vi "Grab.vi"() -> ()   [LabVIEW 2013]
doc: "The Grab VI acquires images continuously and displays the images in an image control using high-level acquisition VIs. A grab is appropriate for high-speed applications in which you need to process only one image at a time."
uses:
  <vilib>/vision/driver/NI_Vision_Acquisition_Software.lvlib
panel:
  out "appended path":path
  in  "Camera Name":refnum<k21> caption="IMAQdx Session"
  out "Buffer Number":u32
  out "Image":T1(plugin-control)
  out "Frame Rate":dbl(knob) scale=0.0..100.0
  in  "Stop":bool
  # "Overview: Demonstrates how to acquire images continuously using a Grab acquisition.\nRequirements: Vision Acquisition Software\nInstructions: \n1. Select the Camera Name.\n2. Run the VI"
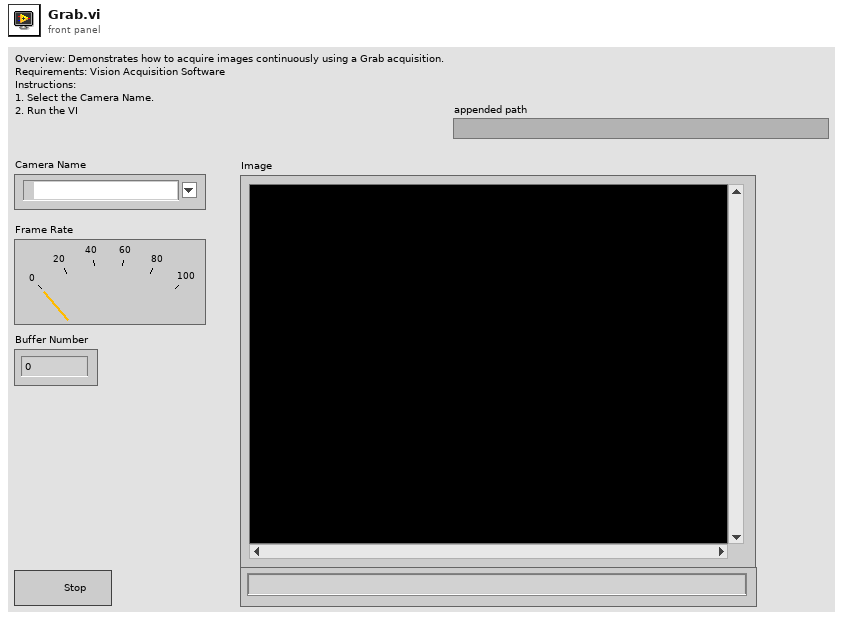
[diagram p1: front panel]
types:
  T1 = typedef "IMAQ Image.ctl" = refnum<image>
  T2 = typedef "IMAQdx.ctl" = refnum<k21>
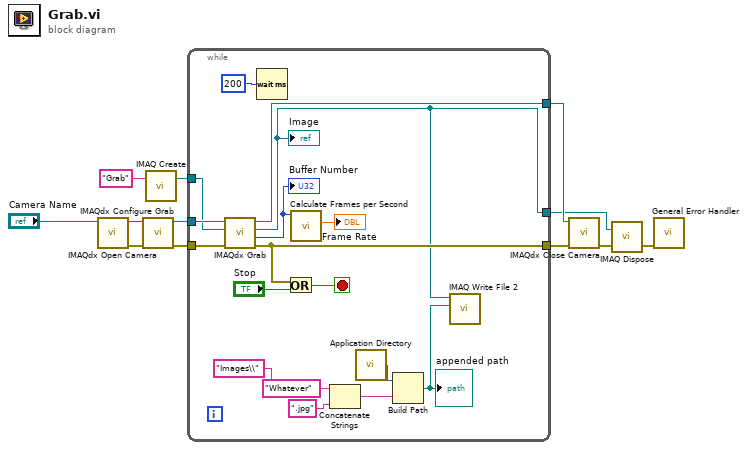
[diagram p0: block diagram]
diagram:
  n1 = call <vilib>:"IMAQdx Open Camera.vi"("Session In"="Camera Name") -> ("error out"=w7:errorcluster, "Session Out"=w6:T2)  [unwired: 2 in, 7 out]
  n2 = call <vilib>:"IMAQdx Configure Grab.vi"("error in"=w7, "Session In"=w6) -> ("error out"=w10:errorcluster, "Session Out"=w11:T2)  [unwired: 8 out]
  n3 = call "IMAQ Create"("Image Name"="Grab") -> ("New Image"=w12:T1)  [unwired: 3 in, 2 out]
  n4 = while {
    tunnel: [w24] -> w9
    tunnel: w10 -> [w26]
    tunnel: w11 -> [w27]
    tunnel: [w21] -> w8
    tunnel: w12 -> [w25]
    tunnel: [w20] -> w4
    stop <- w29 stop-if-true
    n5 = call <vilib>:"IMAQdx Grab.vi"("error in"=w26, "Image In"=w25, "Session In"=w27) -> ("error out"=w21:errorcluster, "Buffer Number Out"=w22:u32, "Image Out"=w20:T1, "Session Out"=w24:T2)  [unwired: 1 in, 4 out]
    "Image" <- w20
    "Buffer Number" <- w22
    n6 = Wait (ms)(milliseconds to wait=u32 200) -> ()  [unwired: 1 out]
    n7 = Or(x=w21, y="Stop") -> (x .or. y?=w29:bool)
    n8 = call <vilib>:"Calculate Frames per Second.vi"("Buffer Number"=w22) -> ("Processed Frames/s"=→"Frame Rate":dbl)  [unwired: 8 in, 2 out]
    n9 = Concatenate Strings("Images\\" ("name or relative path"), "Whatever" ("string"), ".jpg" ("string")) -> (w17:string)
    n10 = call <vilib>:"Application Directory.vi"() -> ("Application Directory"=w19:path)
    n11 = Build Path(base path=w19, name or relative path=w17) -> (appended path=w14:path)
    "appended path" <- w14
    n12 = call-poly "IMAQ Write File 2"("File Path"=w14, "Image"=w20) -> ()  [unwired: 8 in, 2 out]
  }
  n13 = call <vilib>:"IMAQdx Close Camera.vi"("error in"=w8, "Session In"=w9) -> ("error out"=w3:errorcluster)  [unwired: 9 out]
  n14 = call "IMAQ Dispose"("Image"=w4, "error in (no error)"=w3) -> ("error out"=w2:errorcluster)  [unwired: 4 in]
  n15 = call <vilib>:"General Error Handler.vi"("error in (no error)"=w2) -> ()  [unwired: 1 in, 14 out]
